vi "Move Target Manually.vi"(8 "error in (no error)":errorcluster, 10 "Target Speed & Direction":i16=128, 11 "MWWL Verification in":refnum<class "MWWL Verification.lvclass">) -> (0 "error out":errorcluster, 3 "MWWL Verification out":refnum<class "MWWL Verification.lvclass">)   [LabVIEW 2018, in "MWWL Verification.lvlib" / "MWWL Verification.lvclass"]
uses:
  MWWL Verification.lvclass
  MWWL Verification.lvclass/MWWL Verification.ctl
  Range Controller Actor/Range Controller Actor Messages/Move or Stop Range Target Msg/Move or Stop Range Target Msg.lvclass
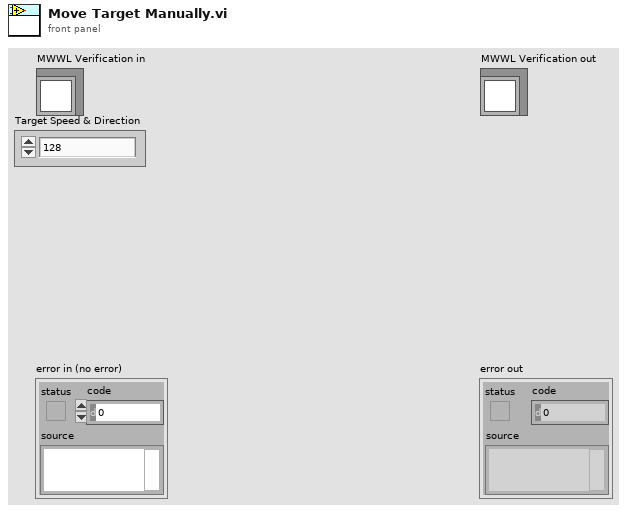
[diagram p1: front panel]
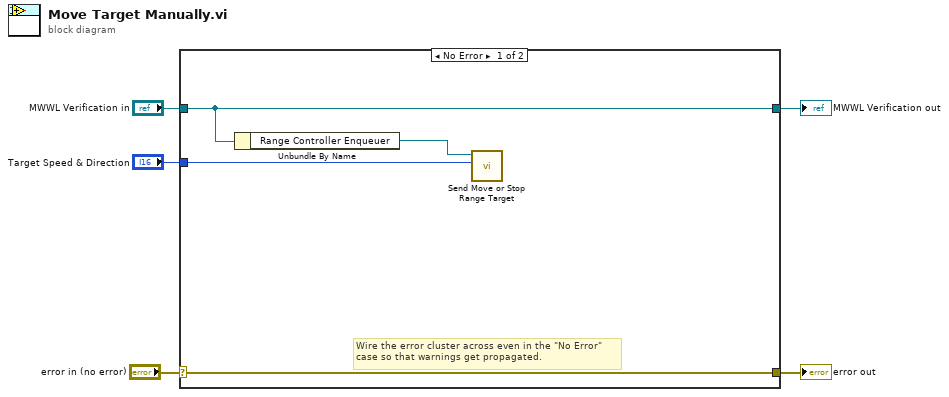
[diagram p0: block diagram]
diagram:
  n1 = case shown="No Error" "error in (no error)" {
    selector: "error in (no error)" -> [w9 w11]
    tunnel: [w9 w11] -> w4
    tunnel: [w8 w10] -> w2
    tunnel: "MWWL Verification in" -> [w8 w10]
    tunnel: "Target Speed & Direction" -> [w6 _]
    frame No Error {
      # "Wire the error cluster across even in the \"No Error\"\ncase so that warnings get propagated."
      n2 = Unbundle By Name(w8) -> ("Range Controller Enqueuer"=w7:refnum<class "Message Enqueuer.lvclass">)
      n3 = call "Send Move or Stop Range Target.vi"("Target Speed & Direction"=w6, "Message Enqueuer in"=w7) -> ()  [unwired: 8 in, 2 out]
    }
    frame Error {
    }
  }
  "error out" <- w4
  "MWWL Verification out" <- w2
